vi "Write Trace Payload.vi"(8 "error in (no error)":errorcluster, 10 "Trace Payload":string, 11 "Trace in":refnum<class "Trace.lvclass">) -> (0 "error out":errorcluster, 3 "Trace out":refnum<class "Trace.lvclass">)   [LabVIEW 2014, in "Robot Actor Framework.lvlib" / "Trace.lvlib" / "Trace.lvclass"]
uses:
  Trace.lvclass
  Trace.lvclass/Trace.ctl
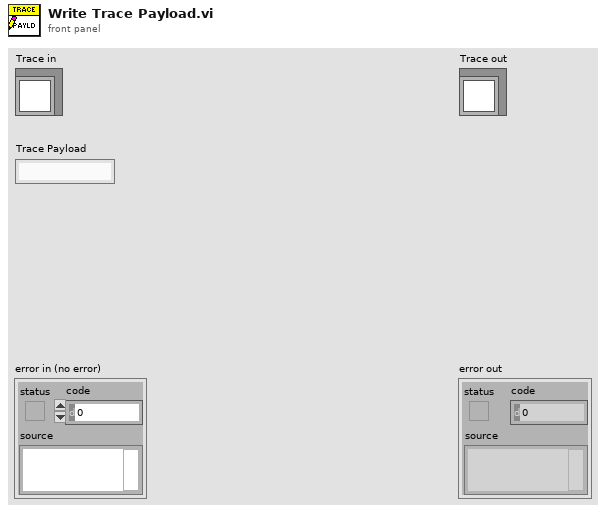
[diagram p1: front panel]
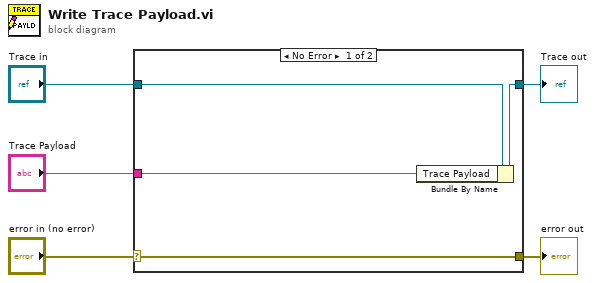
[diagram p0: block diagram]
diagram:
  n1 = case shown="No Error" "error in (no error)" {
    selector: "error in (no error)" -> [w9 w10]
    tunnel: [w9 w10] -> w4
    tunnel: [w7 w11] -> w2
    tunnel: "Trace in" -> [w8 w11]
    tunnel: "Trace Payload" -> [w6 _]
    frame No Error {
      n2 = Bundle By Name(cluster=w8, "Trace Payload"=w6) -> (w7:refnum<class "Trace.lvclass">)
    }
    frame Error {
    }
  }
  "error out" <- w4
  "Trace out" <- w2
